vi "SR430_bins_2_bins_per_record.vi"(2 "bins":i32, 5 "error in (no error)":errorcluster) -> (16 "binPerRecord":i32, 17 "In Range?":bool, 19 "error out":errorcluster)   [LabVIEW 2009, in "SR430Driver.lvlib"]
doc: "Converts the number of bins per record in user friendly format into the number of bins per record into the format as used by the instrument. Intermdiate values are rounded to the next higher value number. The instruments supports up to 16384 bins per record in steps of 1024 bins.\n\nVI Tree for the SR430 Multi-Channel Scaler from Staford Research Systems.\n\nHistory: 24-APR-2002, Dietrich Beck\n\nCopyright (C)\nGesellschaft für Schwerionenforschung, GSI\nPlanckstr. 1\n64291 Darmstadt\nGermany\n\nContact: D.Beck@gsi.de \n\nThis program is free software; you can redistribute it and/or modify it under the terms of the \nGNU General Public License as published by the Free Software Foundation; either version 2 of the license, or (at your option) any later version.\n\nThis program is distributed in the hope that it will be useful, but WITHOUT ANY WARRANTY; without even the implied warranty of MERCHANTABILITY or FITNESS FOR A PARTICULAR PURPOSE. See the GNU General License for more details (http://www.gnu.org).\n\nGesellschaft für Schwerionenforschung, GSI\nPlanckstr. 1, 64291 Darmstadt, Germany\nFor all questions and ideas contact: M.Richter@gsi.de, K.Poppensieker, H.Brand@gsi.de or D.Beck@gsi.de.\nLast update: 11-APR-2002"
uses:
  SR430Driver.lvlib
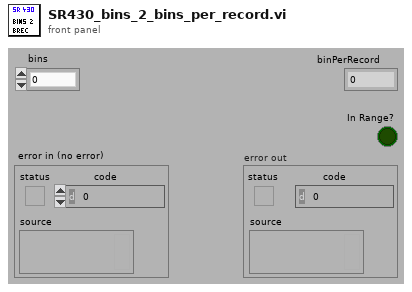
[diagram p1: front panel]
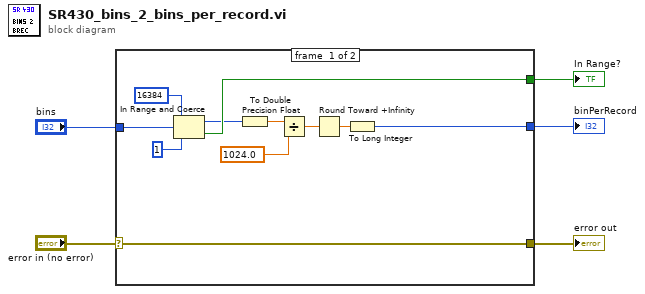
[diagram p0: block diagram]
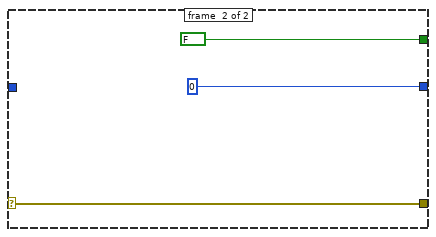
[diagram p2: hidden frame]
diagram:
  n1 = case shown="No Error" "error in (no error)" {
    selector: "error in (no error)" -> [w16 w19]
    tunnel: [w16 w19] -> w4
    tunnel: "bins" -> [w15 _]
    tunnel: [w6 0] -> w2
    tunnel: [w12 FALSE] -> w1
    frame #0 {
      n2 = In Range and Coerce(upper limit=16384, x=w15, lower limit=1) -> (coerced(x)=w11:i32, In Range?=w12:bool)
      n3 = To Double Precision Float(number=w11) -> (double precision float=w10:dbl)
      n4 = Divide(x=w10, y=1024.0) -> (x/y=w8:dbl)
      n5 = Round Toward +Infinity ("Round To +Infinity")(x=w8) -> (ceil(x): smallest int >= x=w7:dbl)
      n6 = To Long Integer(number=w7) -> (32bit integer=w6:i32)
    }
    frame #1 {
    }
  }
  "error out" <- w4
  "binPerRecord" <- w2
  "In Range?" <- w1
